vi "List Compatible Ctls.vi"(11 "ValueUIP In":refnum<class "ValueUIP.lvclass">) -> (2 "Compatible Ctl Classes":string[](array[string]), 3 "ValueUIP Out":refnum<class "ValueUIP.lvclass">)   [LabVIEW 2015, in "ValueUIP.lvclass"]
doc: "Overwrite this method in your child UIPs to provide a custom list of VI Server Control Classes compatible with that UIP."
uses:
  ValueUIP.lvclass
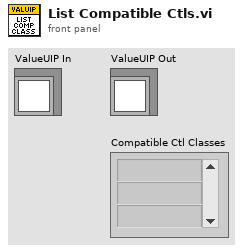
[diagram p1: front panel]
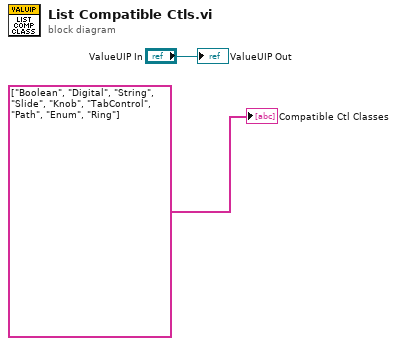
[diagram p0: block diagram]
diagram:
  "Compatible Ctl Classes" <- string[] ["Boolean", "Digital", "String", "Slide", "Knob", "TabControl", "Path", "Enum", "Ring"]
  "ValueUIP Out" <- "ValueUIP In"
